vi "Reset_Instr.vi"(8 "error in (no error)":errorcluster caption="entrée d'erreur (pas d'erreur)", 11 "Class DIO en entrée":refnum<class "Class Instrument DIO.lvclass">) -> (0 "error out":errorcluster caption="sortie d'erreur", 3 "Class DIO en Sortie":refnum<class "Class Instrument DIO.lvclass">)   [LabVIEW 2020, in "Library Instrument & Equipement.lvlib" / "Library Instruments.lvlib" / "Class Instrument DIO.lvclass"]
uses:
  Class Instrument DIO.lvclass
  Class Instrument DIO.lvclass/Class Instrument DIO.ctl
  Instrument (Default)/Class Instrument (Default).lvclass
  DIO/Class DIO (Default)/Class DIO (Default).lvclass
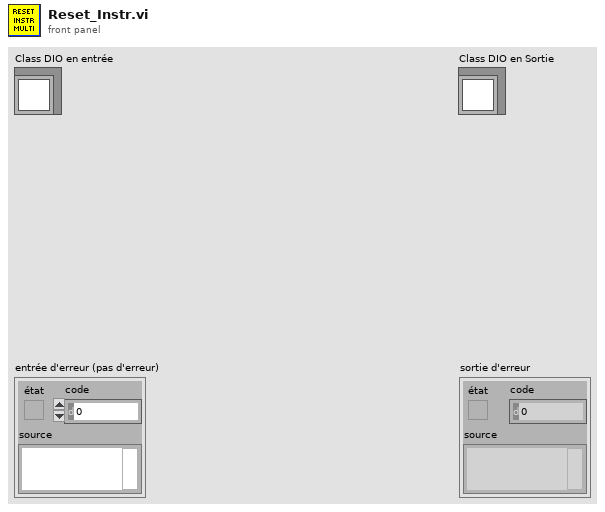
[diagram p1: front panel]
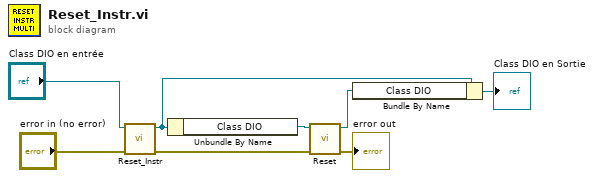
[diagram p0: block diagram]
diagram:
  n1 = call-parent "Reset_Instr.vi"("error in (no error)"="error in (no error)", "Class Instrument (Default) en entrée"="Class DIO en entrée") -> ("error out"=w4:errorcluster, "Class Instrument (Default) en sortie"=w5:refnum<class "Class Instrument DIO.lvclass">)  [unwired: 8 in]
  n2 = Unbundle By Name(w5) -> ("Class DIO"=w2:refnum<class "Class DIO (Default).lvclass">)
  n3 = call-dynamic "Reset.vi"("error in (no error)"=w4, "Class DIO (Default) en entrée"=w2) -> ("error out"=→"error out":errorcluster, "Class DIO (Default) en sortie"=w1:refnum<class "Class DIO (Default).lvclass">)  [unwired: 8 in]
  n4 = Bundle By Name(cluster=w5, "Class DIO"=w1) -> (→"Class DIO en Sortie":refnum<class "Class Instrument DIO.lvclass">)
